vi "(SubVI) Set Gain.vi"(4 "error in (no error)":errorcluster, 6 "Gain":dbl(slide) scale=0.0..23.9 scale format="%#.1f", 7 "Refnum in":T1) -> (0 "error out":errorcluster, 2 "Gain read":dbl, 3 "Refnum out":T1)   [LabVIEW 2014]
uses:
  <vilib>/userdefined/High Color/IMAQdx.ctl
  <resource>/objmgr/imaqdx.rc
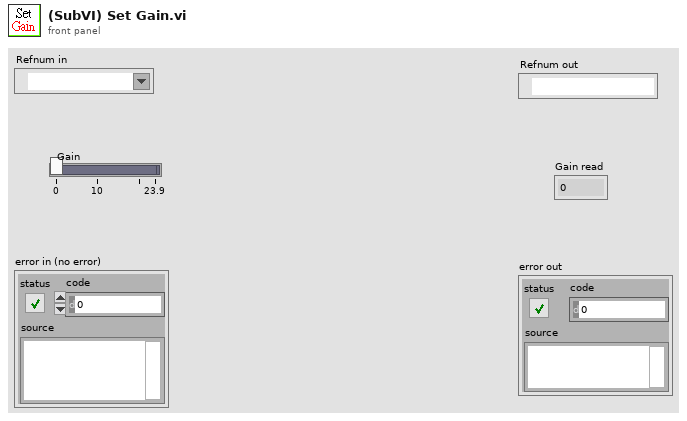
[diagram p1: front panel]
types:
  T1 = typedef "IMAQdx.ctl" = refnum<k21>
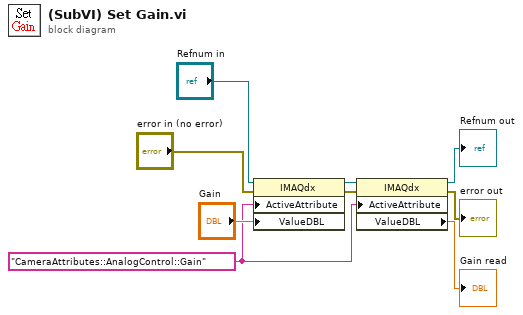
[diagram p0: block diagram]
diagram:
  w2 = "CameraAttributes::AnalogControl::Gain"
  n1 = property class="IMAQdx"(reference="Refnum in", error in="error in (no error)", "ActiveAttribute"=w2, "ValueDBL"="Gain") -> (reference out=w4:T1, error out=w3:errorcluster)
  n2 = property class="IMAQdx"(reference=w4, error in=w3, "ActiveAttribute"=w2) -> (reference out=→"Refnum out":T1, error out=→"error out":errorcluster, "ValueDBL"=→"Gain read":dbl)
